vi "Raise or Lower Abort.vi"(8 "error in (no error)":errorcluster, 9 "Sender":string, 10 "New Abort Value":bool, 11 "Guardian in":refnum<class "Guardian.lvclass">) -> (0 "error out":errorcluster, 3 "Guardian out":refnum<class "Guardian.lvclass">)   [LabVIEW 2026, in "TALOS.lvlib" / "Guardian.lvlib" / "Guardian.lvclass"]
uses:
  Guardian.lvclass
  C:/LabVIEW Code/TALOS/talos/Ancestor/Ancestor/Ancestor.lvclass
  C:/LabVIEW Code/TALOS/builds/Actor Framework PPL/Actor Framework.lvlibp/1abvi3w/vi.lib/ActorFramework/Actor/Actor.lvclass
  Guardian.lvclass/Guardian.ctl
  Abort Processing actions.ctl
  Ancestor/Ancestor/Ancestor.lvclass/Ancestor.ctl
  builds/Actor Framework PPL/Actor Framework.lvlibp/1abvi3w/vi.lib/ActorFramework/Message Enqueuer/Message Priority.ctl
  Guardian Messages/Message to Other Guardian Msg/Message to Other Guardian Msg.lvclass/Message to Other Guardian Msg.ctl
  Guardian Messages/TCP-SV Message Interpreter Msg/TCP-SV Message Interpreter Msg.lvclass/TCP-SV Message Interpreter Msg.ctl
  Guardian Messages/Message to Other Guardian Msg/Send Message to Other Guardian.vi
  Support VIs/Search Array of Strings.vi
  Guardian Messages/TCP-SV Message Interpreter Msg/Send TCP-SV Message Interpreter.vi
  Support VIs/Generate Error.vi
  FGV/Error Memory/Get Error Description.vi
  Support VIs/Get PC name.vi
  Support VIs/Get Class Name.vi
  <vilib>/Utility/error.llb/Clear Errors.vi
  FGV/Error Memory/Error Memory Core.vi
  <vilib>/AdvancedString/Delimited String to 1D String Array.vi
  <vilib>/AdvancedString/Delimited String to 1D String Array (string).vi
  Support VIs/Circus Root Path.vi
  FGV/Error Memory/Error Crt Lvl checker.vi
  FGV/Error Memory/Error Memory Core.vi/40c8088d-b597-4017-91af-faa98e00292e.vi
  FGV/Error Memory/Error Memory Core.vi/d4a3ab98-063c-4e44-b43d-fbdcfe6c2be2.vi
  Pat message.vi
  Support VIs/Global Constants.vi
  Support VIs/Circus Critical PCs List.vi
  builds/Actor Framework PPL/Actor Framework.lvlibp/1abvi3w/vi.lib/ActorFramework/Actor/Read Self Enqueuer.vi
  builds/Actor Framework PPL/Actor Framework.lvlibp/1abvi3w/vi.lib/ActorFramework/Message Enqueuer/Enqueue.vi
  Support VIs/Global Memory.vi
  <vilib>/Utility/LVClass/Get LV Class Name.vi
  Support VIs/Is in Packed Library.vi
  Support VIs/TALOS Root path.vi
  Support VIs/Read CSV worksheet.vi
  <vilib>/Utility/error.llb/General Error Handler.vi
  Support VIs/Error Log.vi
  Guardian Messages/Message to Other Guardian Msg/Message to Other Guardian Msg.lvclass
  Guardian Messages/TCP-SV Message Interpreter Msg/TCP-SV Message Interpreter Msg.lvclass
  Ancestor/Ancestor/Ancestor.lvclass
  <vilib>/Comparison/Equal/Equal Functor/Equal Functor.lvclass
  Classes/Guardian List/Guardian List.lvclass
  builds/Actor Framework PPL/Actor Framework.lvlibp/1abvi3w/vi.lib/ActorFramework/Message Enqueuer/Message Enqueuer.lvclass
  TALOS.lvlib
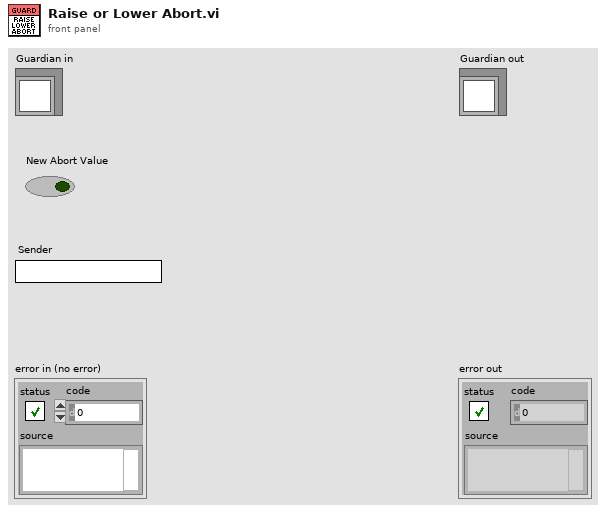
[diagram p1: front panel]
types:
  T1 = typedef "TALOS.lvlib/Guardian.lvlib/Guardian.lvclass/Abort Processing actions.ctl" = enum16{"Propagate locally", "Send to all CIRCUS", "Send to Bearer", "Ignore"}
  T2 = typedef "Actor Framework.lvlibp/Message Enqueuer.lvclass/Message Priority.ctl" = enum16{"Low", "Normal", "High"}
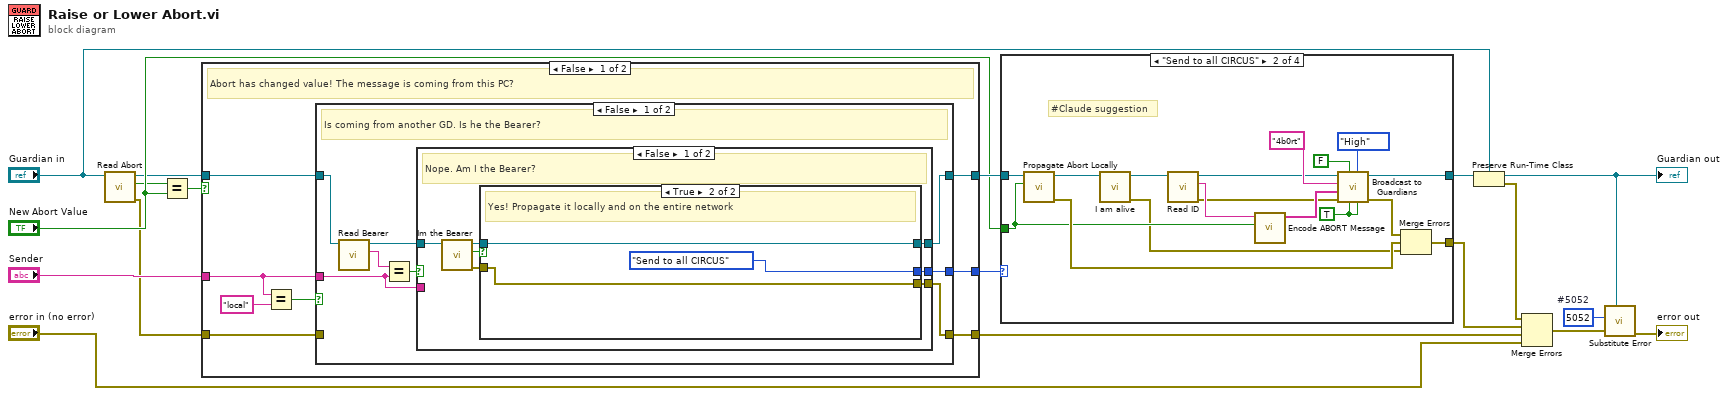
[diagram p0: block diagram]
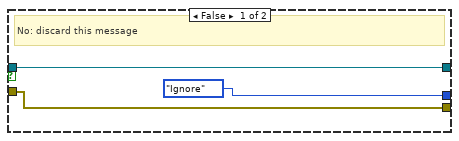
[diagram p2: hidden frame]
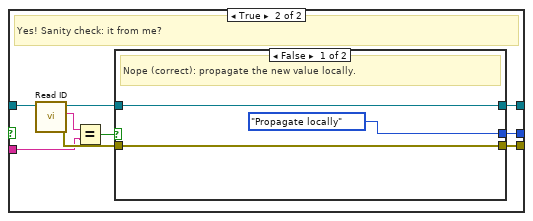
[diagram p3: hidden frame]
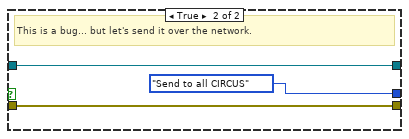
[diagram p4: hidden frame]
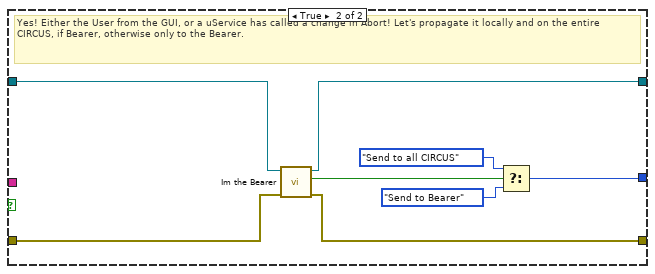
[diagram p5: hidden frame]
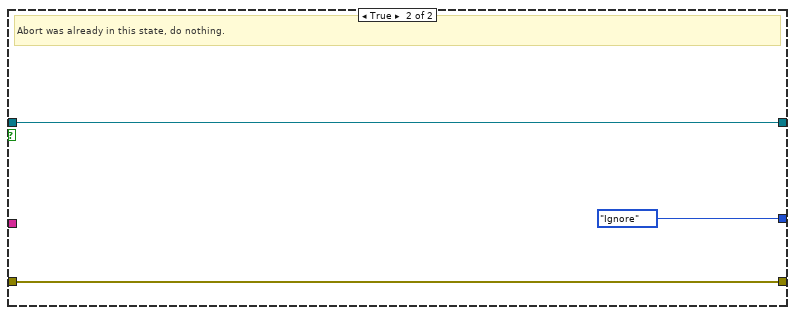
[diagram p6: hidden frame]
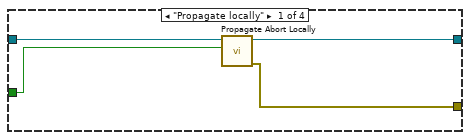
[diagram p7: hidden frame]
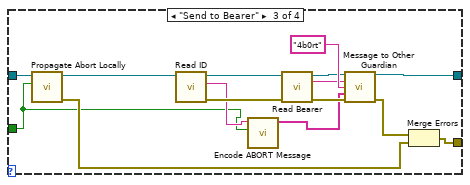
[diagram p8: hidden frame]
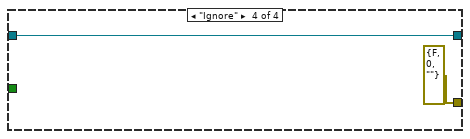
[diagram p9: hidden frame]
diagram:
  w6 = 5052  # #5052
  n1 = call "Read Abort.vi"("Guardian in"="Guardian in") -> ("error out"=w1:errorcluster, "Abort"=w2:bool, "Guardian out"=w4:refnum<class "Guardian.lvclass">)  [unwired: 8 in]
  n2 = Equal?(x=w2, y="New Abort Value") -> (x = y?=w16:bool)
  n3 = case shown="False" w16 {
    tunnel: w4 -> [w25 w73]
    tunnel: [w22 w73] -> w15
    tunnel: w1 -> [w23 w72]
    tunnel: [w20 w72] -> w18
    tunnel: "Sender" -> [w21 _]
    tunnel: [w19 Abort_Processing_actions."Ignore"] -> w13
    frame False {
      # "Abort has changed value! The message is coming from this PC?"
      n4 = Equal?(x=w21, y="local") -> (x = y?=w24:bool)
      n5 = case shown="False" w24 {
        tunnel: w25 -> [w34 w70]
        tunnel: w23 -> [_ w68]
        tunnel: [w29 w67] -> w22
        tunnel: w21 -> [w27 _]
        tunnel: [w30 w69] -> w20
        tunnel: [w28 w64] -> w19
        frame False {
          # "Is coming from another GD. Is he the Bearer?"
          n6 = call "Read Bearer.vi"("Guardian in"=w34) -> ("Bearer"=w33:string, "Guardian out"=w31:refnum<class "Guardian.lvclass">)  [unwired: 8 in, 1 out]
          n7 = Equal?(x=w33, y=w27) -> (x = y?=w32:bool)
          n8 = case shown="False" w32 {
            tunnel: w31 -> [w41 w55]
            tunnel: [w36 w48] -> w30
            tunnel: [w37 w50] -> w29
            tunnel: [w35 w49] -> w28
            tunnel: w27 -> [_ w53]
            frame False {
              # "Nope. Am I the Bearer?"
              n9 = call "Im the Bearer.vi"("Guardian in"=w41) -> ("error out"=w38:errorcluster, "I'm the Bearer"=w40:bool, "Guardian out"=w39:refnum<class "Guardian.lvclass">)  [unwired: 8 in]
              n10 = case shown="True" w40 {
                tunnel: w39 -> [w44 w47]
                tunnel: w38 -> [w43 w46]
                tunnel: [w44 w47] -> w37
                tunnel: [w43 w46] -> w36
                tunnel: [Abort_Processing_actions."Ignore" Abort_Processing_actions."Send to all CIRCUS"] -> w35
                frame False {
                  # "No: discard this message"
                }
                frame True {
                  # "Yes! Propagate it locally and on the entire network"
                }
              }
            }
            frame True {
              # "Yes! Sanity check: it from me?"
              n11 = call "Read ID.vi"("Ancestor in"=w55) -> ("error out"=w56:errorcluster, "ID"=w54:string, "Ancestor out"=w51:refnum<class "Guardian.lvclass">)  [unwired: 8 in]
              n12 = Equal?(x=w54, y=w53) -> (x = y?=w52:bool)
              n13 = case shown="False" w52 {
                tunnel: w51 -> [w59 w62]
                tunnel: [w59 w62] -> w50
                tunnel: [Abort_Processing_actions."Propagate locally" Abort_Processing_actions."Send to all CIRCUS"] -> w49
                tunnel: w56 -> [w57 w60]
                tunnel: [w57 w60] -> w48
                frame False {
                  # "Nope (correct): propagate the new value locally."
                }
                frame True {
                  # "This is a bug... but let's send it over the network."
                }
              }
            }
          }
        }
        frame True {
          # "Yes! Either the User from the GUI, or a uService has called a change in Abort! Let's propagate it locally and on the entire CIRCUS, if Bearer, otherwise only to the Bearer."
          n14 = call "Im the Bearer.vi"("error in (no error)"=w68, "Guardian in"=w70) -> ("error out"=w69:errorcluster, "I'm the Bearer"=w63:bool, "Guardian out"=w67:refnum<class "Guardian.lvclass">)  [unwired: 7 in]
          n15 = Select(t=Abort_Processing_actions."Send to all CIRCUS", s=w63, f=Abort_Processing_actions."Send to Bearer") -> (s? t:f=w64:T1)
        }
      }
    }
    frame True {
      # "Abort was already in this state, do nothing."
    }
  }
  n16 = case shown="\"Send to all CIRCUS\"" w13 {
    tunnel: w15 -> [w76 w87 w103 w111]
    tunnel: [w75 w85 w101 w111] -> w14
    tunnel: "New Abort Value" -> [w74 w84 w95 _]
    tunnel: [w77 w86 w102 errorcluster {"status"=FALSE, "code"=0, "source"=""} ("error IO")] -> w11
    frame "Propagate locally" {
      n17 = call "Propagate Abort Locally.vi"("New Abort Value"=w74, "Guardian in"=w76) -> ("error out"=w77:errorcluster, "Guardian out"=w75:refnum<class "Guardian.lvclass">)  [unwired: 8 in]
    }
    frame "Send to all CIRCUS" {
      w81 = TRUE ("Only active ones?")
      # "#Claude suggestion"
      n18 = call "Propagate Abort Locally.vi"("New Abort Value"=w84, "Guardian in"=w87) -> ("error out"=w93:errorcluster, "Guardian out"=w80:refnum<class "Guardian.lvclass">)  [unwired: 8 in]
      n19 = call "I am alive.vi"("Guardian in"=w80) -> ("error out"=w78:errorcluster, "Guardian out"=w79:refnum<class "Guardian.lvclass">)  [unwired: 9 in]
      n20 = call "Read ID.vi"("Ancestor in"=w79) -> ("error out"=w88:errorcluster, "ID"=w92:string, "Ancestor out"=w89:refnum<class "Guardian.lvclass">)  [unwired: 8 in]
      n21 = call "Encode ABORT Message.vi"("Abort"=w84, "Sender ID"=w92) -> ("Abort Message"=w91:string[])  [unwired: 9 in]
      n22 = call "Broadcast to Guardians.vi"("Critical PCs also?"=w81, "Message Priority"=Message_Priority."High", "Only active ones?"=w81, "Local also?"=FALSE, "error in (no error)"=w88, "Data"=w91, "Message"="4b0rt", "Guardian in"=w89) -> ("error out"=w94:errorcluster, "Guardian out"=w85:refnum<class "Guardian.lvclass">)  [unwired: 2 in]
      n23 = Merge Errors(w94, w93, w78) -> (w86:errorcluster)
    }
    frame "Send to Bearer" {
      n24 = call "Propagate Abort Locally.vi"("New Abort Value"=w95, "Guardian in"=w103) -> ("error out"=w107:errorcluster, "Guardian out"=w109:refnum<class "Guardian.lvclass">)  [unwired: 8 in]
      n25 = call "Read ID.vi"("Ancestor in"=w109) -> ("error out"=w104:errorcluster, "ID"=w96:string, "Ancestor out"=w105:refnum<class "Guardian.lvclass">)  [unwired: 8 in]
      n26 = call "Encode ABORT Message.vi"("Abort"=w95, "Sender ID"=w96) -> ("Abort Message"=w97:string[])  [unwired: 9 in]
      n27 = call "Read Bearer.vi"("error in (no error)"=w104, "Guardian in"=w105) -> ("error out"=w99:errorcluster, "Bearer"=w98:string, "Guardian out"=w100:refnum<class "Guardian.lvclass">)  [unwired: 7 in]
      n28 = call "Message to Other Guardian.vi"("Guardian in"=w100, "Guardian ID"=w98, "Message"="4b0rt", "Data"=w97, "error in (no error)"=w99) -> ("Guardian out"=w101:refnum<class "Guardian.lvclass">, "error out"=w108:errorcluster)  [unwired: 9 in]
      n29 = Merge Errors(w108, w107) -> (w102:errorcluster)
    }
    frame "Ignore" {
    }
  }
  n30 = Preserve Run-Time Class(object in=w14, 2:"Guardian in") -> (object out=w7:refnum<class "Guardian.lvclass">, error out=w10:errorcluster)  [unwired: 1 in]
  "Guardian out" <- w7
  n31 = Merge Errors(w10, w11, w18, "error in (no error)") -> (w9:errorcluster)
  n32 = call "Substitute Error.vi"("LabVIEW Object"=w7, "error in (no error)"=w9, "Error Code"=w6) -> ("error out"=→"error out":errorcluster)  [unwired: 8 in]
